vi "Disable Controls TS Safe.vi"(8 "error in (no error)":errorcluster, 10 "Disabled":T1(ring), 11 "Main in":refnum<class "Main.lvclass">) -> (0 "error out":errorcluster, 3 "Main out":refnum<class "Main.lvclass">)   [LabVIEW 2023, in "GUI.lvlib" / "Main.lvlib" / "Main.lvclass"]
uses:
  Main.lvclass
  Main.lvclass/Main.ctl
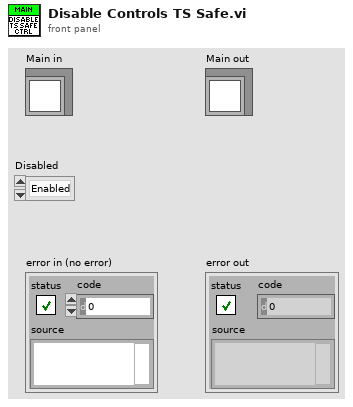
[diagram p1: front panel]
types:
  T1 = enum8{"Enabled", "Disabled", "Disabled and Grayed Out"}
  T2 = typedef "GUI.lvlib/Main.App.Cluster.ctl" = cluster{"Sidebar":refnum<vi>, "Menubar":refnum<vi>, "Log in And Out":refnum<vi>, "User Level":refnum<vi>, "User":refnum<vi>, "Sub Panel":refnum<vi>, "Panel Name":refnum<vi>, "Menu":refnum<vi>, "Close":refnum<vi>}
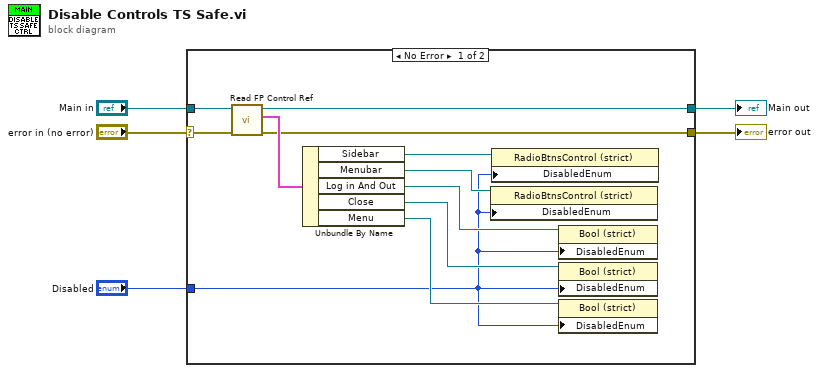
[diagram p0: block diagram]
diagram:
  n1 = case shown="No Error" "error in (no error)" {
    selector: "error in (no error)" -> [w13 w18]
    tunnel: [w12 w18] -> w4
    tunnel: [w14 w17] -> w2
    tunnel: "Main in" -> [w15 w17]
    tunnel: "Disabled" -> [w6 _]
    frame No Error {
      n2 = call "Read FP Control Ref.vi"("error in (no error)"=w13, "Main in"=w15) -> ("error out"=w12:errorcluster, "FP Control Ref"=w16:T2, "Main out"=w14:refnum<class "Main.lvclass">)  [unwired: 7 in]
      n3 = Unbundle By Name(w16) -> ("Sidebar"=w11:refnum<vi>, "Menubar"=w10:refnum<vi>, "Log in And Out"=w9:refnum<vi>, "Close"=w8:refnum<vi>, "Menu"=w7:refnum<vi>)
      n4 = property class="RadioBtnsControl (strict)"(reference=w10, "DisabledEnum"=w6) -> ()  [unwired: 1 in, 2 out]
      n5 = property class="RadioBtnsControl (strict)"(reference=w11, "DisabledEnum"=w6) -> ()  [unwired: 1 in, 2 out]
      n6 = property class="Bool (strict)"(reference=w9, "DisabledEnum"=w6) -> ()  [unwired: 1 in, 2 out]
      n7 = property class="Bool (strict)"(reference=w8, "DisabledEnum"=w6) -> ()  [unwired: 1 in, 2 out]
      n8 = property class="Bool (strict)"(reference=w7, "DisabledEnum"=w6) -> ()  [unwired: 1 in, 2 out]
    }
    frame Error {
    }
  }
  "error out" <- w4
  "Main out" <- w2
